vi "YOLOv5_OpenVINO_IR_NIVision.vi"() -> ()   [LabVIEW 2018]
doc: "YOLOv5_OpenVINO_IR_imgs: This example is an object detection example of the YOLOv5 algorithm, which can achieve object detection function on sample images. IR is OpenVINO's proprietary optimized format model."
uses:
  vi.lib/VIRobotics/ModelZoo/Object_Detection/yolov5_openvino/InitialModel_yolov5_OpenVINO_IR.vi
  vi.lib/VIRobotics/ModelZoo/Object_Detection/yolov5_openvino/yolov5_openvino.lvclass
  <vilib>/vision/driver/NI_Vision_Acquisition_Software.lvlib
panel:
  in  "device_name":string(combo)="CPU"
  in  "bin_fle":path=path "C:/ProgramData/VIRobotics/ModelZoo/Object_Detection/yolov5/IR_model/yolov5s.bin"
  out "每帧耗时(s)":dbl
  in  "Stop":bool
  out "Image":T1(plugin-control)
  in  "Camera Name":refnum<k21>="cam0" caption="IMAQdx Session"
  in  "class_names_file":path=path "C:/ProgramData/VIRobotics/ModelZoo/Object_Detection/coco.names"
  in  "xml_file":path=path "C:/ProgramData/VIRobotics/ModelZoo/Object_Detection/yolov5/IR_model/yolov5s.xml"
  # "Overview: Demonstrates how to use OpenVINO to load the the IR model of yolov5 for real-time object detection.\nRequirements: Windows.\nMake sure your computer has a camera。\nInstructions: \n1.Select the device_name to use.（If your computer has Intel GPU, you can select GPU in the \"type\" control before running the VI to achieve faster inference).\n2.Run the VI.\nIf you want to load the model you trained, follow the following steps:\n1.Select the device_name to use. \n2.Specify the xml_file、bin_file and class_names_file.\n3.Run the VI."
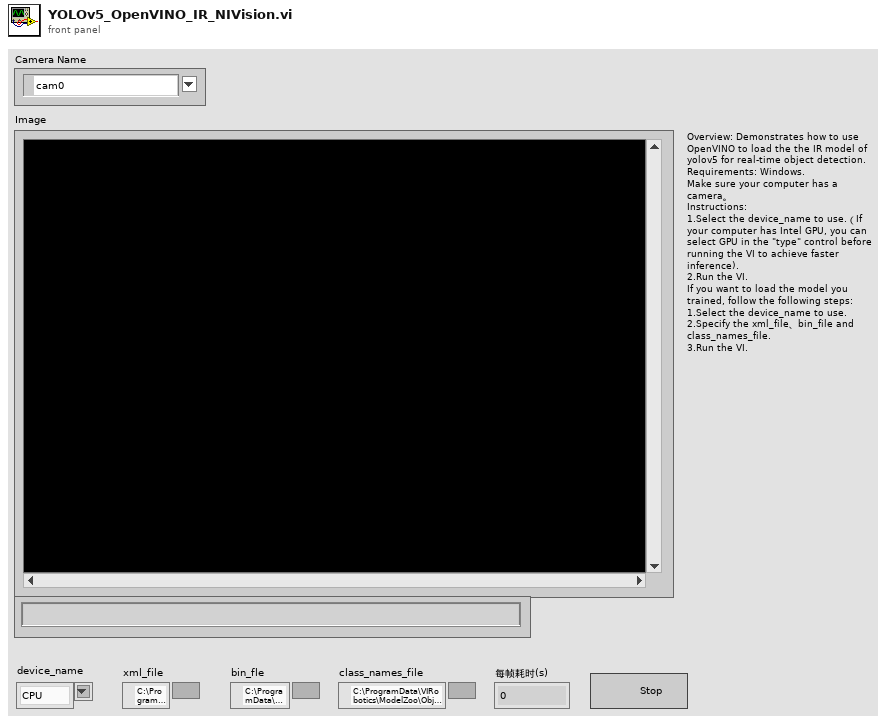
[diagram p1: front panel]
types:
  T1 = typedef "IMAQ Image.ctl" = refnum<image>
  T2 = typedef "IMAQdx.ctl" = refnum<k21>
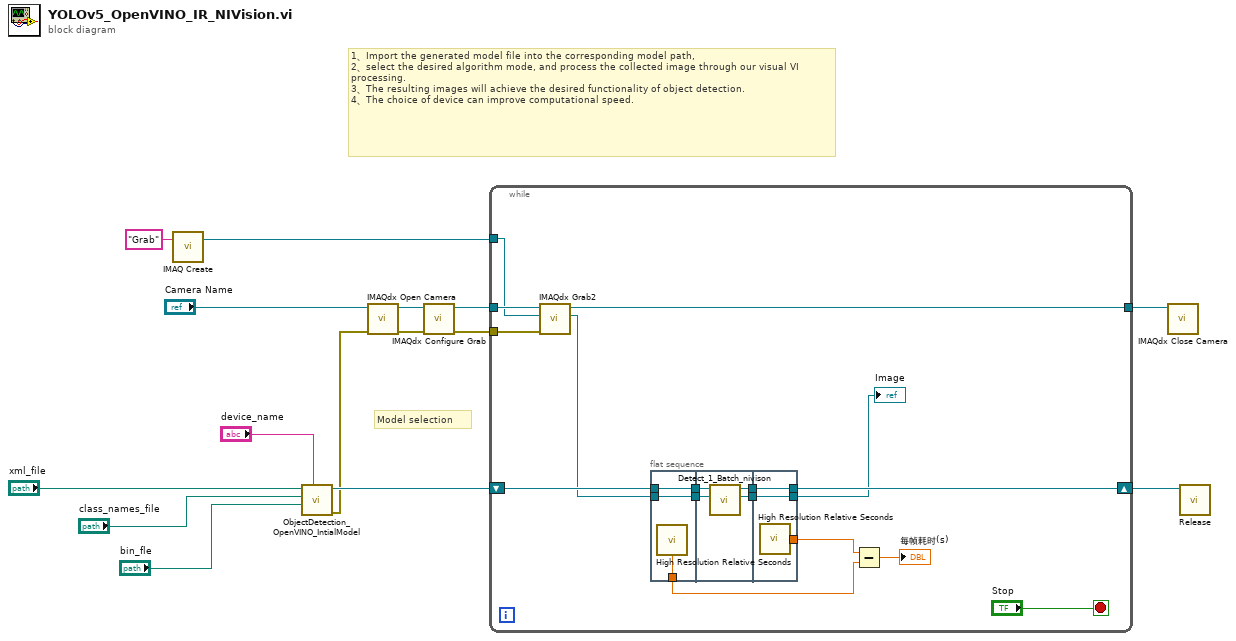
[diagram p0: block diagram]
diagram:
  # "1、Import the generated model file into the corresponding model path, \n2、select the desired algorithm mode, and process the collected image through our visual VI processing. \n3、The resulting images will achieve the desired functionality of object detection. \n4、The choice of device can improve computational speed."
  # "Model selection"
  n1 = call "IMAQ Create"("Image Name"="Grab") -> ("New Image"=w8:T1)  [unwired: 3 in, 2 out]
  n2 = call-poly "ObjectDetection_OpenVINO_IntialModel.vi"("device_name"="device_name", "bin_fle"="bin_fle", "class_names_path"="class_names_file", "xml path"="xml_file") -> ("error out"=w5:errorcluster, "yolov5_openvino out"=w14:refnum<class "yolov5_openvino.lvclass">)  [unwired: 6 in]
  n3 = call <vilib>:"IMAQdx Open Camera.vi"("error in"=w5, "Session In"="Camera Name") -> ("error out"=w13:errorcluster, "Session Out"=w12:T2)  [unwired: 1 in, 7 out]
  n4 = call <vilib>:"IMAQdx Configure Grab.vi"("error in"=w13, "Session In"=w12) -> ("error out"=w6:errorcluster, "Session Out"=w9:T2)  [unwired: 8 out]
  n5 = while {
    shift-right: [w30] -> w15
    shift-left: w14 -> [w31]
    tunnel: w9 -> [w29]
    tunnel: w8 -> [w27]
    tunnel: [w26] -> w7
    tunnel: w6 -> [w25]
    stop <- "Stop" stop-if-true
    n6 = call <vilib>:"IMAQdx Grab2.vi"("error in"=w25, "Image In"=w27, "Session In"=w29) -> ("Image Out"=w24:T1, "Session Out"=w26:T2)  [unwired: 5 in, 2 out]
    n7 = flat-sequence {
      tunnel: w24 -> [w33]
      tunnel: w31 -> [w34]
      tunnel: [w34] -> w20
      tunnel: [w33] -> w19
      tunnel: [w32] -> w18
      tunnel: [w37] -> w22
      tunnel: [w36] -> w21
      tunnel: w20 -> [w38]
      tunnel: w19 -> [w35]
      tunnel: [w40] -> w28
      tunnel: [w41] -> w30
      tunnel: w22 -> [w41]
      tunnel: w21 -> [w40]
      tunnel: [w39] -> w17
      frame #0 {
        n8 = call <vilib>:"High Resolution Relative Seconds.vi"() -> ("relative seconds"=w32:dbl)
      }
      frame #1 {
        n9 = call-dynamic "Detect_1_Batch_nivison.vi"("Image"=w35, "yolov5_openvino in"=w38) -> ("Image out"=w36:T1, "yolov5_openvino out"=w37:refnum<class "yolov5_openvino.lvclass">)  [unwired: 6 in, 2 out]
      }
      frame #2 {
        n10 = call <vilib>:"High Resolution Relative Seconds.vi"() -> ("relative seconds"=w39:dbl)
      }
    }
    n11 = Subtract(x=w17, y=w18) -> (x-y=→"每帧耗时(s)":dbl)
    "Image" <- w28
  }
  n12 = call <vilib>:"IMAQdx Close Camera.vi"("Session In"=w7) -> ()  [unwired: 1 in, 10 out]
  n13 = call-dynamic "Release.vi"("yolov5_openvino in"=w15) -> ()  [unwired: 9 in, 2 out]
